vi "Read Control (by Reference).vi"(8 "error in (no error)":errorcluster, 11 "ctl path":path) -> (0 "error out":errorcluster, 2 "VI Description":string, 3 "Value":variant)   [LabVIEW 2019, in "JSON-Schema.lvlib"]
uses:
  JSON-Schema.lvlib
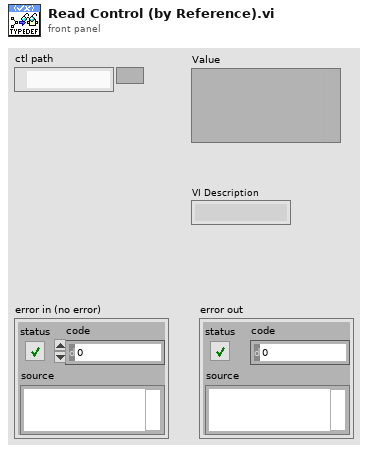
[diagram p1: front panel]
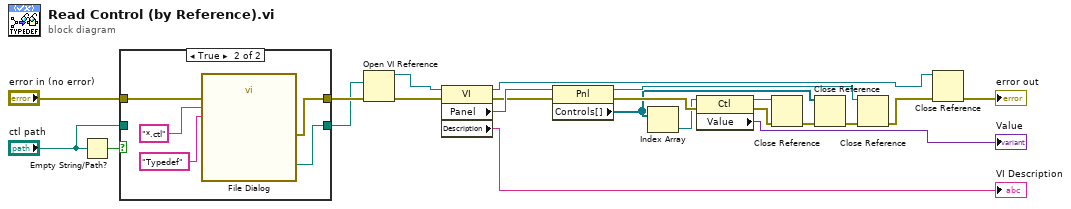
[diagram p0: block diagram]
diagram:
  n1 = Empty String/Path?(string/path="ctl path") -> (empty?=w18:bool)
  n2 = case shown="True" w18 {
    tunnel: [w24 w29] -> w12
    tunnel: "error in (no error)" -> [w23 w28]
    tunnel: [w23 w27] -> w19
    tunnel: "ctl path" -> [w24 _]
    frame False {
    }
    frame True {
      n3 = call "File Dialog"("error in"=w28, "pattern (all files)"="*.ctl", "pattern label"="Typedef") -> ("selected path"=w29:path, "error out"=w27:errorcluster)  [unwired: 9 in, 2 out]
    }
  }
  n4 = Open VI Reference(vi path=w12, error in (no error)=w19) -> (vi reference=w22:refnum<vi>, error out=w21:errorcluster)  [unwired: 4 in]
  n5 = property class="VI"(reference=w22, error in=w21) -> (reference out=w15:refnum<vi>, error out=w1:errorcluster, "Panel"=w2:refnum<vi>, "Description"=→"VI Description":string)
  n6 = property class="Pnl"(reference=w2, error in=w1) -> (reference out=w4:refnum<vi>, error out=w10:errorcluster, "Controls[]"=w3:refnum<vi>[])
  n7 = Index Array(array=w3) -> (element=w5:refnum<vi>)  [unwired: 1 in]
  n8 = property class="Ctl"(reference=w5, error in=w10) -> (reference out=w7:refnum<vi>, error out=w9:errorcluster, "Value"=→"Value":variant)
  n9 = Close Reference(reference=w7, error in (no error)=w9) -> (error out=w8:errorcluster)
  n10 = Close Reference(reference=w3, error in (no error)=w8) -> (error out=w6:errorcluster)
  n11 = Close Reference(reference=w4, error in (no error)=w6) -> (error out=w13:errorcluster)
  n12 = Close Reference(reference=w15, error in (no error)=w13) -> (error out=→"error out":errorcluster)
